vi "Coord window-Update filename ind.vi"(8 "error in (no error)":errorcluster, 9 "File path":path, 11 "File name indicator ref":refnum<vi>) -> (0 "error out":errorcluster)   [LabVIEW 2020]
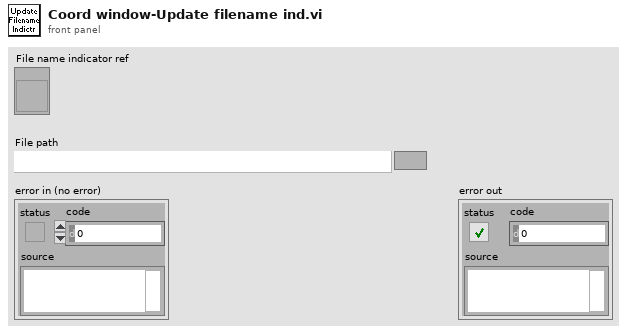
[diagram p1: front panel]
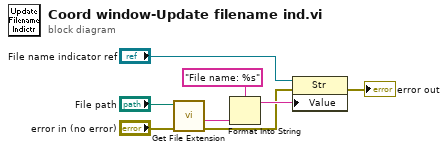
[diagram p0: block diagram]
diagram:
  n1 = call <vilib>:"Get File Extension.vi"("error in (no error)"="error in (no error)", "file"="File path") -> ("error out"=w2:errorcluster, "filename without extension"=w7:string)  [unwired: 5 in, 3 out]
  n2 = Format Into String(format string="File name: %s", w7) -> (resulting string=w8:string)  [unwired: 2 in, 1 out]
  n3 = property on="Property Node" class="Str"(reference="File name indicator ref", error in=w2, "Value"=w8) -> (error out=→"error out":errorcluster)  [unwired: 1 out]
